vi "Get Reference.vi"(8 "error in (no error)":errorcluster, 10 "Numeric":i32, 11 "UI Reference Wrapper in":refnum<class "UI Reference Wrapper.lvclass">) -> (0 "error out":errorcluster, 1 "Name":string, 2 "VI Refnum":refnum<vi>, 3 "UI Reference Wrapper out":refnum<class "UI Reference Wrapper.lvclass">)   [LabVIEW 2020, in "UI Reference Wrapper.lvclass"]
uses:
  UI Reference Wrapper.lvclass
  UI Reference Wrapper.lvclass/UI Reference Wrapper.ctl
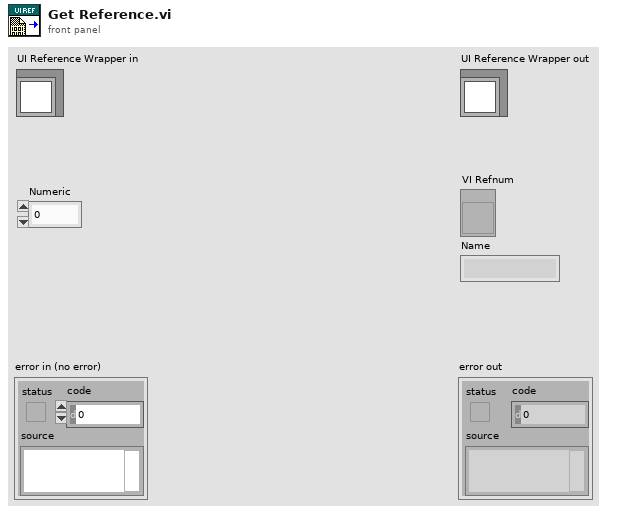
[diagram p1: front panel]
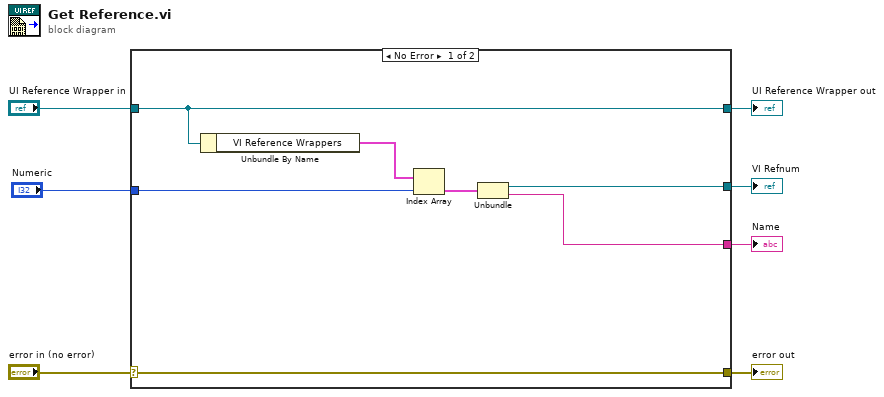
[diagram p0: block diagram]
diagram:
  n1 = case shown="No Error" "error in (no error)" {
    selector: "error in (no error)" -> [w14 w16]
    tunnel: [w14 w16] -> w6
    tunnel: [w13 w15] -> w4
    tunnel: "UI Reference Wrapper in" -> [w13 w15]
    tunnel: "Numeric" -> [w11 _]
    tunnel: [w9 _] -> w2
    tunnel: [w8 _] -> w1
    frame No Error {
      n2 = Unbundle By Name(w13) -> ("VI Reference Wrappers"=w12:cluster{"VI Refnum":refnum<vi>, "Name":string}[])
      n3 = Index Array(array=w12, index=w11) -> (element=w10:cluster{"VI Refnum":refnum<vi>, "Name":string})
      n4 = Unbundle(w10) -> ("VI Refnum"=w9:refnum<vi>, "Name"=w8:string)
    }
    frame Error {
    }
  }
  "error out" <- w6
  "UI Reference Wrapper out" <- w4
  "VI Refnum" <- w2
  "Name" <- w1
